vi "X-Y Graph.vi"() -> ()   [LabVIEW 2012]
doc: "This VI illustrates the various data types that the XY Graph accepts.\n\nUse the XY Graph to display data that is not uniformly distributed along the X-axis. This is particularly useful when displaying data that was sampled at a variable rate.\n\nSee the Waveform Graph.vi for an example of how to use the Waveform Graph.\n\n_KEYWORDS_: graph, XY"
panel:
  out "(X and Y arrays) Multi Plot":cluster{i32[], dbl[]}[](graph)
  out "(X and Y arrays) Single Plot":cluster{i32[], dbl[]}(graph)
  out "(Array of Pts) Multi Plot":cluster{cluster{i32, dbl}[]}[](graph)
  out "(Array of Pts) Single Plot":cluster{i32, dbl}[](graph)
  # "Use the XY Graph to display data that is not uniformly distributed along the X-axis.  This is particularly useful when displaying data that was sampled at a variable rate.  This VI illustrates the various data \ntypes that the XY graph accepts.  Press <ctrl-h> for more information."
  # "Array of Pts"
  # "X and Y arrays"
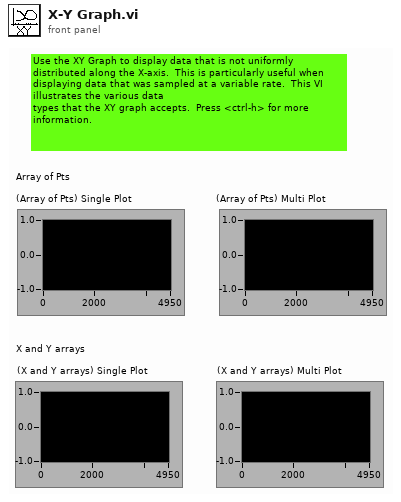
[diagram p1: front panel]
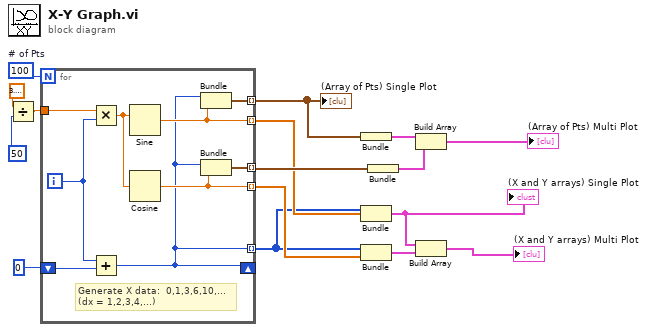
[diagram p0: block diagram]
diagram:
  w16 = 100  # # of Pts
  n1 = Divide(x=3.141592653589793, y=50) -> (x/y=w14:dbl)
  n2 = for {
    N: w16 -> [_]
    tunnel: w14 -> [w24]
    shift-right: [w17] -> _
    shift-left: 0 -> [w25]
    tunnel: [w20] -> w6 mode=indexing
    tunnel: [w21] -> w5 mode=indexing
    tunnel: [w19] -> w12 mode=indexing
    tunnel: [w18] -> w11 mode=indexing
    tunnel: [w17] -> w4 mode=indexing
    i -> [w23]
    # "Generate X data:  0,1,3,6,10,...\n(dx = 1,2,3,4,...)"
    n3 = Multiply(x=w24, y=w23) -> (x*y=w22:dbl)
    n4 = Add(x=w23, y=w25) -> (x+y=w17:i32)
    n5 = Sine(x=w22) -> (sin(x)=w20:dbl)
    n6 = Cosine(x=w22) -> (cos(x)=w21:dbl)
    n7 = Bundle "Bundle"(w17, w20) -> (w19:cluster{i32, dbl})  [unwired: 1 in]
    n8 = Bundle "Bundle"(w17, w21) -> (w18:cluster{i32, dbl})  [unwired: 1 in]
  }
  "(Array of Pts) Single Plot" <- w12
  n9 = Bundle "Bundle"(w12) -> (w9:cluster{cluster{i32, dbl}[]})  [unwired: 1 in]
  n10 = Bundle "Bundle"(w4, w6) -> (w2:cluster{i32[], dbl[]})  [unwired: 1 in]
  "(X and Y arrays) Single Plot" <- w2
  n11 = Bundle "Bundle"(w4, w5) -> (w3:cluster{i32[], dbl[]})  [unwired: 1 in]
  n12 = Bundle(w11) -> (w10:cluster{cluster{i32, dbl}[]})  [unwired: 1 in]
  n13 = Build Array "Build Array"(w9, w10) -> (→"(Array of Pts) Multi Plot":cluster{cluster{i32, dbl}[]}[])
  n14 = Build Array "Build Array"(w2, w3) -> (→"(X and Y arrays) Multi Plot":cluster{i32[], dbl[]}[])
